vi "Parse Header.vi"(10 "Header":string, 11 "IPersist in":refnum<class "IPersist.lvclass">) -> (1 "Value":string[](array[string]), 2 "Name":string[](array[string]), 3 "IPersist out":refnum<class "IPersist.lvclass">)   [LabVIEW 2020, in "IPersist.lvlib" / "IPersist.lvclass"]
uses:
  <vilib>/gpm_packages/@cs/persistence/source/IPersist/IPersist.lvclass
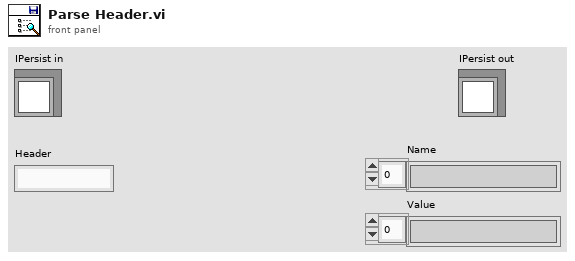
[diagram p1: front panel]
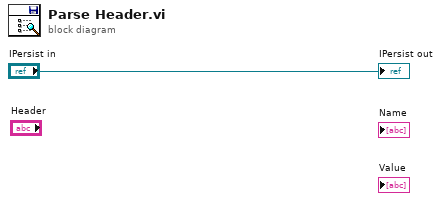
[diagram p0: block diagram]
diagram:
  "IPersist out" <- "IPersist in"
